vi "Periodic Tasks.vi"(8 "error in":errorcluster) -> ()   [LabVIEW 2016]
doc: "This VI runs in parallel to other tasks. It can contain as many user-defined periodic loops as you need. These can carry out PID or other sorts of timed response."
uses:
  <vilib>/Rock Robotics/WPI/Utilities/WPI_GetSetVariantRefNum.vi
  Robot Global Data.vi
  NavX Library/NavX/NavX Library.lvlib
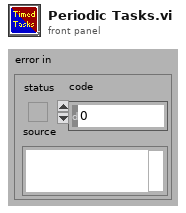
[diagram p1: front panel]
types:
  T1 = typedef "WPI_EncoderDevRef.ctl" = cluster{"DevStatus":errorcluster, "EncoderIndex":T2, "CounterIndex":T3, "DistancePerCount":dbl, "Decoding Type":T4}
  T2 = typedef "FPGA_EncoderIdx.ctl" = enum8{"Enc 0", "Enc 1", "Enc 2", "Enc 3", "Enc 4", "Enc 5", "Enc 6", "Enc 7", "Invalid"}
  T3 = typedef "FPGA_CounterCtrSystemIndex.ctl" = enum8{"Ctr 0", "Ctr 1", "Ctr 2", "Ctr 3", "Ctr 4", "Ctr 5", "Ctr 6", "Ctr 7", "Invalid"}
  T4 = typedef "WPI_EncoderType.ctl" = enum16{"1x", "2x", "4x"}
  T5 = typedef "WPI_RobotDriveDevRef.ctl" = cluster{"DevStatus":errorcluster, "Motors[]":T6[], "Square Inputs":bool, "Max Output":dbl}
  T6 = typedef "WPI_MotorControlDeviceRef.ctl" = cluster{"DeviceStatus":errorcluster, "Type":T7, "PWM":cluster{"PWM Channel":T8, "DeadBand":T9}, "CAN":cluster{"Device Number":u8, "SetOutput VI Ref":variant, "GetOutput VI Ref":variant, "Enable VI Ref":variant, "Disable VI Ref":variant, "Data":variant}, "Invert":bool}
  T7 = typedef "WPI_MotorControlType.ctl" = enum16{"PWM", "CAN"}
  T8 = typedef "FPGA_DIOPWMChannel.ctl" = enum8{"PWM 0", "PWM 1", "PWM 2", "PWM 3", "PWM 4", "PWM 5", "PWM 6", "PWM 7", "PWM 8", "PWM 9", "PWM MXP 0", "PWM MXP 1", "PWM MXP 2", "PWM MXP 3", "PWM MXP 4", "PWM MXP 5", "PWM MXP 6", "PWM MXP 7", "PWM MXP 8", "PWM MXP 9", "Invalid"}
  T9 = typedef "WPI_PWMDeadband.ctl" = cluster{"Name":string, "maxPositivePwm":i32, "minPositivePwm":i32, "centerPwm":i32, "maxNegativePwm":i32, "minNegativePwm":i32, "angularRange":u16}
  T10 = cluster{"Yaw":dbl, "Roll":dbl, "Pitch":dbl, "Heading":dbl, "Fused Heading":dbl}
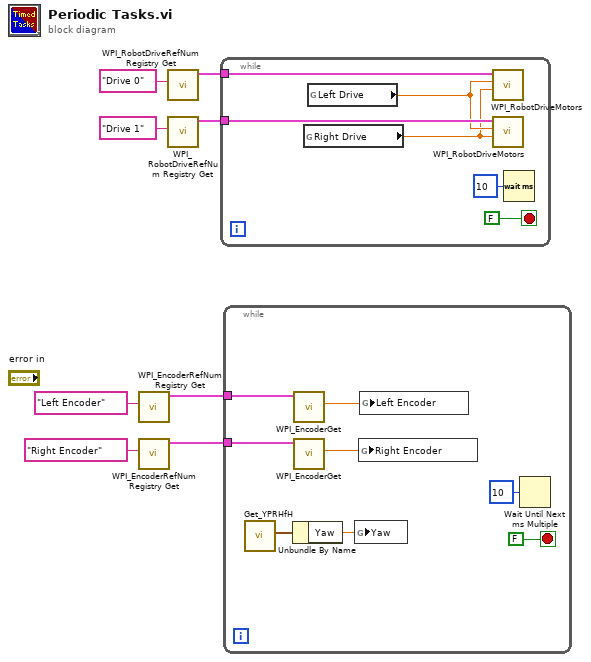
[diagram p0: block diagram]
diagram:
  n1 = call <vilib>:"WPI_EncoderRefNum Registry Get.vi"("refnum name"="Left Encoder") -> ("EncoderDevRef"=w2:T1)  [unwired: 9 in, 1 out]
  n2 = call <vilib>:"WPI_EncoderRefNum Registry Get.vi"("refnum name"="Right Encoder") -> ("EncoderDevRef"=w1:T1)  [unwired: 9 in, 1 out]
  n3 = call <vilib>:"WPI_RobotDriveRefNum Registry Get.vi"("refnum name"="Drive 0") -> ("RobotDriveDevRef"=w5:T5)  [unwired: 9 in, 1 out]
  n4 = call <vilib>:"WPI_RobotDriveRefNum Registry Get.vi"("refnum name"="Drive 1") -> ("RobotDriveDevRef"=w6:T5)  [unwired: 9 in, 1 out]
  n5 = while {
    tunnel: w6 -> [w11]
    tunnel: w5 -> [w12]
    stop <- FALSE stop-if-true
    n6 = global read "Robot Global Data.vi" "Right Drive"() -> (w9:dbl)
    n7 = global read "Robot Global Data.vi" "Left Drive"() -> (w10:dbl)
    n8 = call <vilib>:"WPI_RobotDriveMotors.vi"("RightSpeed"=w9, "LeftSpeed"=w10, "RobotDriveDevRef"=w12) -> ()  [unwired: 6 in, 3 out]
    n9 = call <vilib>:"WPI_RobotDriveMotors.vi"("RightSpeed"=w9, "LeftSpeed"=w10, "RobotDriveDevRef"=w11) -> ()  [unwired: 6 in, 3 out]
    n10 = Wait (ms)(milliseconds to wait=u32 10) -> ()  [unwired: 1 out]
  }
  n11 = while {
    tunnel: w2 -> [w20]
    tunnel: w1 -> [w19]
    stop <- FALSE stop-if-true
    n12 = call "Get_YPRHfH.vi"() -> ("YRPHfH"=w15:T10)  [unwired: 11 in]
    n13 = Unbundle By Name(w15) -> ("Yaw"=w16:dbl)
    n14 = call <vilib>:"WPI_EncoderGet.vi"("EncoderDevRef"=w20) -> ("Distance"=w18:dbl)  [unwired: 5 in, 5 out]
    n15 = call <vilib>:"WPI_EncoderGet.vi"("EncoderDevRef"=w19) -> ("Distance"=w17:dbl)  [unwired: 5 in, 5 out]
    n16 = global write "Robot Global Data.vi" "Yaw"(w16) -> ()
    n17 = global write "Robot Global Data.vi" "Right Encoder"(w17) -> ()
    n18 = global write "Robot Global Data.vi" "Left Encoder"(w18) -> ()
    n19 = Wait Until Next ms Multiple(millisecond multiple=u32 10 ("milliseconds to wait")) -> ()  [unwired: 1 out]
  }
